vi "convert_to_fp.vi"(1 "Input Array":u16[](array[numeric])) -> (0 "Floating point":sgl)   [LabVIEW 2011]
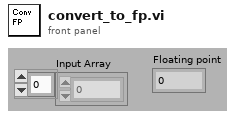
[diagram p1: front panel]
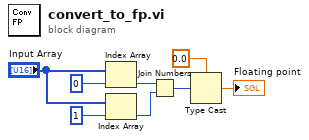
[diagram p0: block diagram]
diagram:
  n1 = Index Array(array="Input Array", index=0) -> (element=w6:u16)
  n2 = Index Array(array="Input Array", index=1) -> (element=w5:u16)
  n3 = Join Numbers(hi=w6, lo=w5) -> ((hi.lo)=w4:u32)
  n4 = Type Cast(type=sgl 0.0, x=w4) -> (*(type *) &x=→"Floating point":sgl)
